vi "Test Geometry Location Fitting Cpp.vi"() -> ()   [LabVIEW 2011]
uses:
  <vilib>/gmath/statdist.llb/Normal Random.vi
  <vilib>/gmath/NI_Gmath.lvlib
  gVision.lvlib
panel:
  out "error out":errorcluster
  out "orthoganality":dbl format="%_4e"
  out "residual":dbl format="%_4e"
  out "orientation":cluster{"pitch":dbl, "roll":dbl, "yaw":dbl} {"pitch" format="%_4e"; "roll" format="%_4e"; "yaw" format="%_4e"}
  out "offset":cluster{"x":dbl, "y":dbl, "z":dbl} {"x" format="%_4e"; "y" format="%_4e"; "z" format="%_4e"}
  in  "Scale\n(mm)":dbl=100.0
  in  "Offset\n(mm)":cluster{"x":dbl, "y":dbl, "z":dbl}
  in  "Orientation\n(degrees)":cluster{"pitch":dbl, "roll":dbl, "yaw":dbl}={"pitch"=0.5, "roll"=0.0, "yaw"=0.0}
  in  "Noise\n(mm)":dbl=10.0
  in  "Sample Size":u32=1000
  # "Fitted Values"
  # "Input Values"
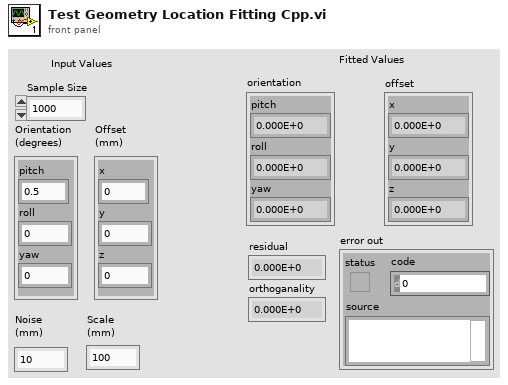
[diagram p1: front panel]
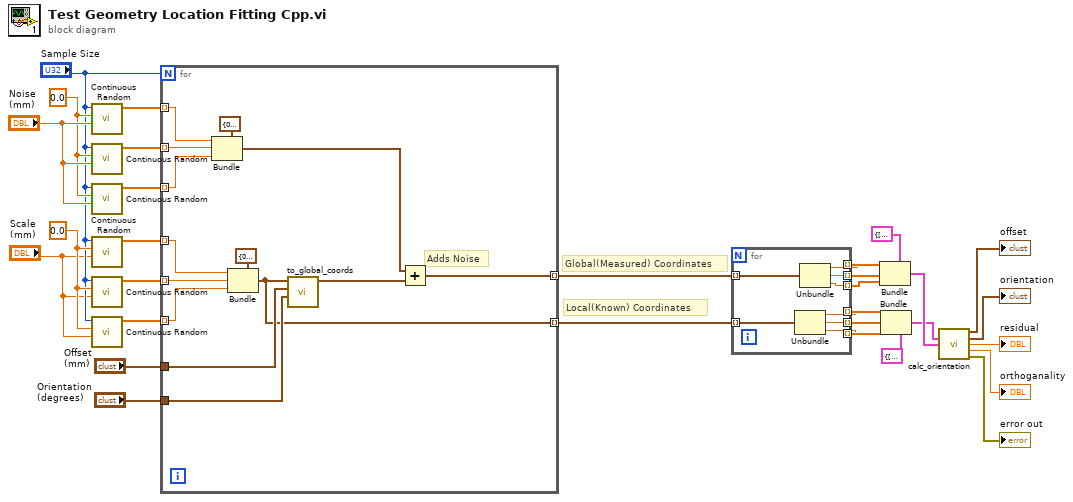
[diagram p0: block diagram]
diagram:
  w25 = 0.0 ("mean")
  w28 = 0.0 ("mean")
  # "Local(Known) Coordinates"
  # "Global(Measured) Coordinates"
  n1 = call-poly <vilib>:"Continuous Random.vi"("std"="Noise\n(mm)", "mean"=w28, "samples"="Sample Size") -> ("normal random data"=w30:dbl[])  [unwired: 7 in, 1 out]
  n2 = call-poly <vilib>:"Continuous Random.vi"("std"="Noise\n(mm)", "mean"=w28, "samples"="Sample Size") -> ("normal random data"=w27:dbl[])  [unwired: 7 in, 1 out]
  n3 = call-poly <vilib>:"Continuous Random.vi"("std"="Noise\n(mm)", "mean"=w28, "samples"="Sample Size") -> ("normal random data"=w26:dbl[])  [unwired: 7 in, 1 out]
  n4 = call-poly <vilib>:"Continuous Random.vi"("std"="Scale\n(mm)", "mean"=w25, "samples"="Sample Size") -> ("normal random data"=w22:dbl[])  [unwired: 7 in, 1 out]
  n5 = call-poly <vilib>:"Continuous Random.vi"("std"="Scale\n(mm)", "mean"=w25, "samples"="Sample Size") -> ("normal random data"=w21:dbl[])  [unwired: 7 in, 1 out]
  n6 = call-poly <vilib>:"Continuous Random.vi"("std"="Scale\n(mm)", "mean"=w25, "samples"="Sample Size") -> ("normal random data"=w20:dbl[])  [unwired: 7 in, 1 out]
  n7 = for {
    N: "Sample Size" -> [_]
    tunnel: w30 -> [w37] mode=indexing
    tunnel: w27 -> [w36] mode=indexing
    tunnel: w26 -> [w35] mode=indexing
    tunnel: w22 -> [w41] mode=indexing
    tunnel: w21 -> [w40] mode=indexing
    tunnel: w20 -> [w39] mode=indexing
    tunnel: "Offset\n(mm)" -> [w43]
    tunnel: "Orientation\n(degrees)" -> [w44]
    tunnel: [w32] -> w17 mode=indexing
    tunnel: [w31] -> w16 mode=indexing
    # "Adds Noise"
    n8 = Bundle(cluster=cluster{"x":dbl, "y":dbl, "z":dbl} {"x"=0.0, "y"=0.0, "z"=0.0} ("local"), "x"=w37, "y"=w36, "z"=w35) -> (w34:cluster{"x":dbl, "y":dbl, "z":dbl})
    n9 = Bundle(cluster=cluster{"x":dbl, "y":dbl, "z":dbl} {"x"=0.0, "y"=0.0, "z"=0.0} ("local"), "x"=w41, "y"=w40, "z"=w39) -> (w31:cluster{"x":dbl, "y":dbl, "z":dbl})
    n10 = call "to_global_coords.vi"("orientation"=w44, "offset"=w43, "local"=w31) -> ("global"=w33:cluster{"x":dbl, "y":dbl, "z":dbl})  [unwired: 7 in, 1 out]
    n11 = Add(x=w34, y=w33) -> (x+y=w32:cluster{"x":dbl, "y":dbl, "z":dbl})
  }
  n12 = for {
    tunnel: w17 -> [w52] mode=indexing
    tunnel: w16 -> [w48] mode=indexing
    tunnel: [w51] -> w14 mode=indexing
    tunnel: [w50] -> w13 mode=indexing
    tunnel: [w49] -> w12 mode=indexing
    tunnel: [w47] -> w10 mode=indexing
    tunnel: [w46] -> w9 mode=indexing
    tunnel: [w45] -> w8 mode=indexing
    n13 = Unbundle(w48) -> ("x"=w47:dbl, "y"=w46:dbl, "z"=w45:dbl)
    n14 = Unbundle(w52) -> ("x"=w51:dbl, "y"=w50:dbl, "z"=w49:dbl)
  }
  n15 = Bundle(cluster=cluster{"x":dbl[], "y":dbl[], "z":dbl[]} {"x"=[], "y"=[], "z"=[]} ("Kx data"), "x"=w14, "y"=w13, "z"=w12) -> (w7:cluster{"x":dbl[], "y":dbl[], "z":dbl[]})
  n16 = Bundle(cluster=cluster{"x":dbl[], "y":dbl[], "z":dbl[]} {"x"=[], "y"=[], "z"=[]} ("Kx data"), "x"=w10, "y"=w9, "z"=w8) -> (w6:cluster{"x":dbl[], "y":dbl[], "z":dbl[]})
  n17 = call "calc_orientation.vi"("Kx data"=w6, "Dx data"=w7) -> ("offset"=→"offset":cluster{"x":dbl, "y":dbl, "z":dbl}, "orientation"=→"orientation":cluster{"pitch":dbl, "roll":dbl, "yaw":dbl}, "residual"=→"residual":dbl, "orthoganality"=→"orthoganality":dbl, "error out"=→"error out":errorcluster)  [unwired: 9 in]
